vi "hextoasc.vi"(11 "HEX输入":string="21") -> (3 "ASCII输出":string)   [LabVIEW 2022 SP3]
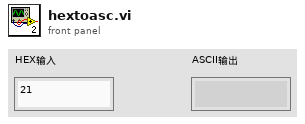
[diagram p1: front panel]
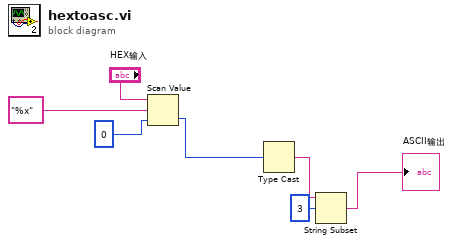
[diagram p0: block diagram]
diagram:
  n1 = Scan Value(string="HEX输入", format string="%x" ("格式字符串"), default (0 dbl)=0) -> (value=w4:i32)  [unwired: 1 out]
  n2 = Type Cast(x=w4) -> (*(type *) &x=w3:string)  [unwired: 1 in]
  n3 = String Subset(string=w3, offset (0)=3 ("偏移量(0)")) -> (substring=→"ASCII输出":string)  [unwired: 1 in]
